vi "Synthesize.vi"(0 "Tone in":refnum<class "Tone.lvclass">, 5 "Fs (Hz)":dbl, 7 "Npts":i32, 9 "Repetition":i32, 11 "error in (no error)":errorcluster) -> (4 "Tone out":refnum<class "Tone.lvclass">, 8 "Array":dbl[](array[numeric]), 15 "error out":errorcluster)   [LabVIEW 2020, in "Tone.lvclass"]
uses:
  Tone.lvclass
  Tone.lvclass/Tone.ctl
  <vilib>/Analysis/NI_AALBase.lvlib
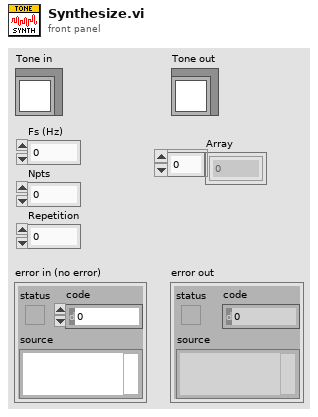
[diagram p1: front panel]
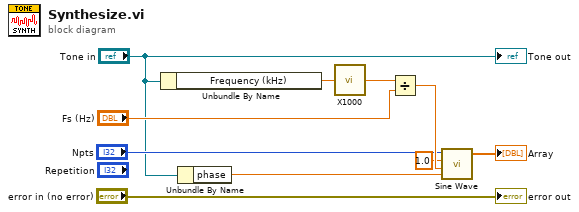
[diagram p0: block diagram]
diagram:
  n1 = Unbundle By Name("Tone in") -> ("Frequency (kHz)"=w8:dbl)
  n2 = Unbundle By Name("Tone in") -> ("phase"=w2:dbl)
  n3 = call "X1000.vi"("X"=w8) -> ("X/1000"=w6:dbl)
  n4 = Divide(x=w6, y="Fs (Hz)") -> (x/y=w10:dbl)
  n5 = call <vilib>:"Sine Wave.vi"("samples"="Npts", "amplitude"=1.0, "frequency"=w10, "phase in"=w2) -> ("sine wave"=→"Array":dbl[])  [unwired: 1 in, 2 out]
  "error out" <- "error in (no error)"
  "Tone out" <- "Tone in"
